vi "All LINX VIs.vi"   [LabVIEW 2020]
uses:
  LabVIEW/vi.lib/MakerHub/LINX/LMH-LINX.lvlib
  LabVIEW/vi.lib/MakerHub/LINX/Public/Utilities/Open TCP.vi
  LabVIEW/vi.lib/MakerHub/LINX/Public/Utilities/Open Local.vi
  LabVIEW/vi.lib/MakerHub/LINX/Public/Utilities/Open Serial.vi
types:
  T1 = typedef "LMH-LINX.lvlib/LINX Ref.ctl" = cluster{"IO":T2, "Interface":T3, "LINX Device Config":T4}
  T2 = typedef "LMH-LINX.lvlib/Platform.ctl" = enum16{"Remote", "Local"}
  T3 = typedef "LMH-LINX.lvlib/Interface.ctl" = enum16{"Serial", "TCP"}
  T4 = typedef "Device.lvlib/LINX Device Config.ctl" = cluster{"Interface":T3, "COM Port":refnum<visa-resource-name>, "TCP Configuration":T5, "Device Family":u8, "Device ID":u8, "Device Name":string, "TCP Ref":refnum<k5>, "Channels":T6}
  T5 = typedef "Device.lvlib/TCP Config.ctl" = cluster{"IP Address":string, "Port":u16}
  T6 = typedef "LMH-LINX.lvlib/Channels.ctl" = cluster{"DI":u8[], "DO":u8[], "AI":u8[], "AO":u8[], "PWM":u8[], "QE":u8[], "UART":u8[], "I2C 2":u8[], "SPI":u8[], "CAN":u8[], "Servo":u8[], "AI Ref (V)":dbl, "AI Resolution (Bits)":u8, "AO Ref (V)":dbl, "AO Resolution (Bits)":u8}
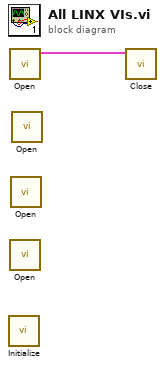
[diagram p0: block diagram]
diagram:
  n1 = call "Initialize.vi"() -> ()  [unwired: 9 in, 3 out]
  n2 = call-poly "Open.vi"() -> ("LINX Resource"=w1:T1)  [unwired: 9 in, 2 out]
  n3 = call-poly "Open.vi"() -> ()  [unwired: 9 in, 3 out]
  n4 = call-poly "Open.vi"() -> ()  [unwired: 9 in, 3 out]
  n5 = call-poly "Open.vi"() -> ()  [unwired: 9 in, 3 out]
  n6 = call "Close.vi"("LINX Resource"=w1) -> ()  [unwired: 10 in, 1 out]
